vi "usrp_stream_rx.vi"() -> ()   [LabVIEW 2014]
uses:
  <vilib>/addons/Modulation/Analog/support/mod_Set Error Source.vi
  <vilib>/addons/Modulation/Digital/Support/Common/Validators/mod_Generate Filter Coefficients Validate.vi
  <vilib>/addons/Modulation/Digital/General/subVIs/mod_Generate Filter Coefficients.vi
  <vilib>/imath/engines/lvmath2/RunTimeEngine/NodeEndStatement/NIMS_NodeEndStatement_Output.vi
  <instcachedir>/0/NIMS_NodeEndStatement_Output_53EC0D466D134D7ABD903AC30B43404B.lvgen/NIMS_NodeEndStatement_Output_53EC0D466D134D7ABD903AC30B43404B_001.vi
  <vilib>/imath/engines/lvmath2/RunTimeEngine/ErrorHandling/NIMS_Finalize Error.vi
  <instrlib>/niUSRP/niUSRP Fetch Rx Data (CDB Cluster).vi
  <vilib>/addons/Modulation/niDMT.lvlib
panel:
  out "error out":errorcluster
  in  "DPSK arity":enum16{"binary", "quadrature"}(ring)=enum."quadrature"
  in  "loop bandwidth":dbl=0.0314
  in  "nfilts":i32=32
  in  "pulse shaping samples per symbol (4)":i32=4
  out "Constellation Graph":cdb[](graph)
  in  "number of samples":i64=20000
  in  "stop":bool
  in  "Timebase Clock Source":string(combo)="Internal"
  in  "Frequency Source":string(combo)="Internal"
  in  "Enabled Channels":string(combo)="0"
  in  "Active Channel":string="0"
  out "coerced gain":dbl=10.0 format="%#_6f"
  out "coerced carrier frequency":dbl=915000000.0 format="%#_6p"
  out "coerced IQ rate":dbl=1000000.0 format="%#_6p"
  in  "active antenna":string="RX2"
  in  "gain":dbl=10.0 format="%#_6f"
  in  "carrier frequency":dbl=915000000.0 format="%#_6p"
  in  "IQ rate":dbl=1000000.0 format="%#_6p"
  in  "device names":refnum<k15>="192.168.10.4"
  # "This is a usrp point-to-point communication link prototype\ndeveloped by Teng-Hui Huang, \nNetwork Information and Communications Laboratory, NTU Taiwan\nThis is the receiver program for USRP streaming mode\n\nQuick start:\n1. Connect USRPs to PC\n2. Run \"usrp_stream_tx.vi\"\n3. Run \"usrp_stream_rx.vi\"\n\nIf no error occur, you will see DPSK symbols on constellation graph\nFor any issues, please send me an e-mail\nhui811116@outlook.com\n\nThanks\nTeng-Hui Huang."
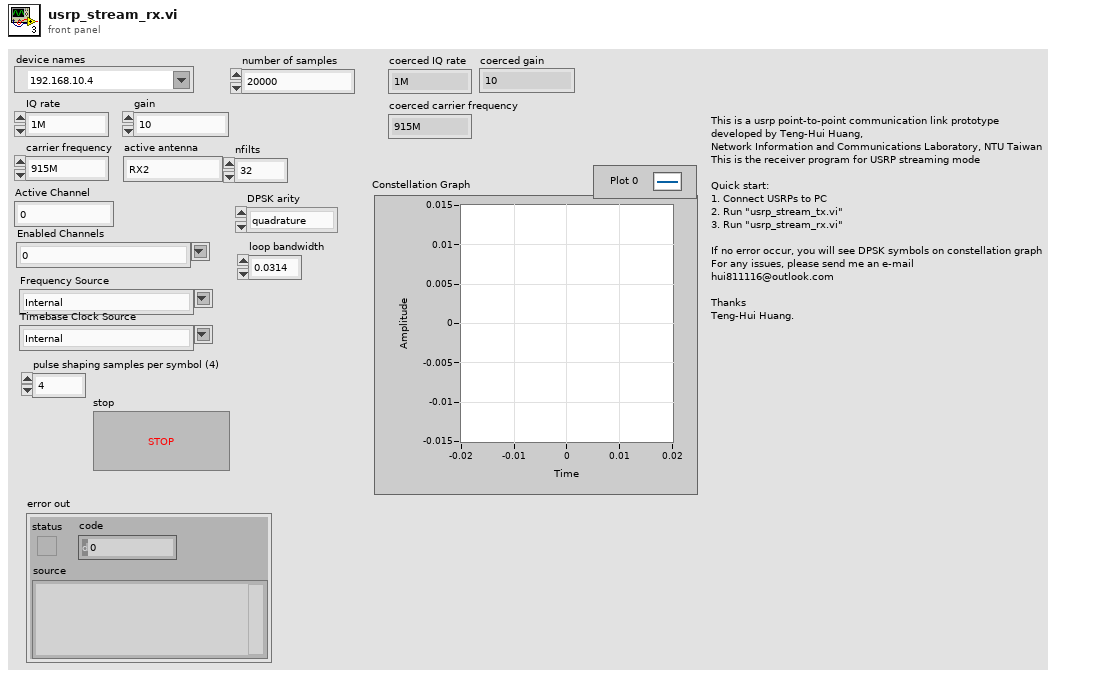
[diagram p1: front panel]
types:
  T1 = enum16{"none", "Raised Cosine", "Root Raised Cos", "Gaussian"}
  T2 = enum16{"FSK", "PSK", "QAM", "MSK", "PAM", "ASK", "CPM"}
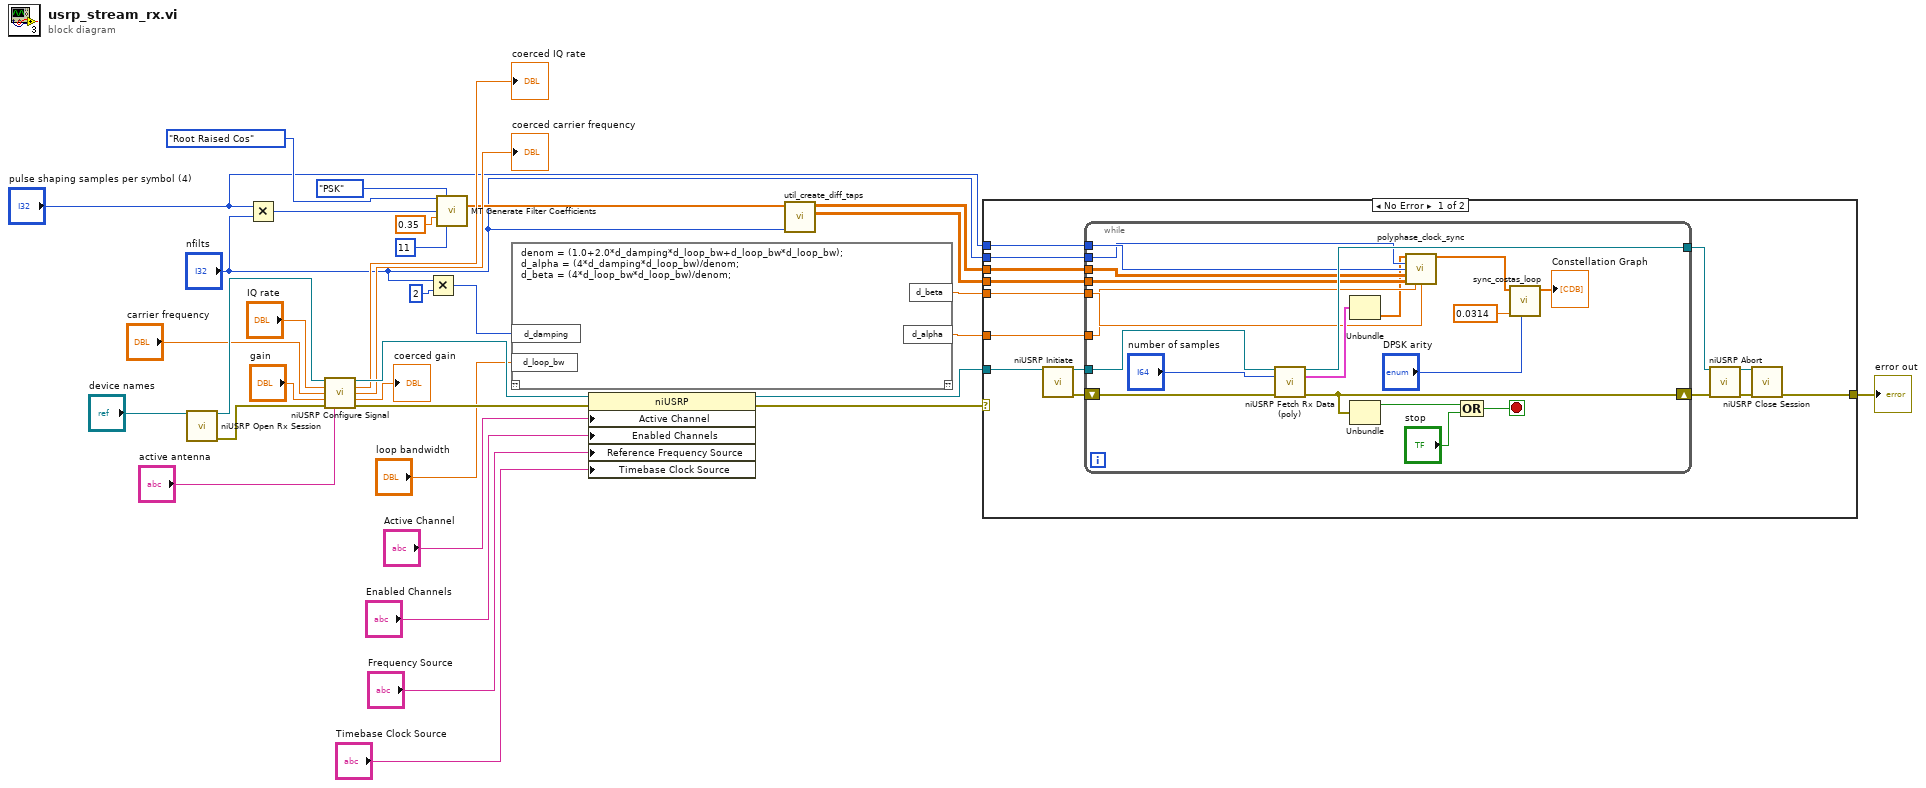
[diagram p0: block diagram]
diagram:
  n1 = call <instrlib>:"niUSRP Open Rx Session.vi"("device names"="device names") -> ("session handle out"=w31:refnum<k15>, "error out"=w30:errorcluster)  [unwired: 13 in]
  n2 = Multiply(x="pulse shaping samples per symbol (4)", y="nfilts") -> (x*y=w2:i32)
  n3 = call <instrlib>:"niUSRP Configure Signal.vi"("session handle"=w31, "IQ rate"="IQ rate", "carrier frequency"="carrier frequency", "gain"="gain", "error in (no error)"=w30, "active antenna"="active antenna") -> ("session handle out"=w33:refnum<k15>, "coerced IQ rate"=→"coerced IQ rate":dbl, "coerced carrier frequency"=→"coerced carrier frequency":dbl, "coerced gain"=→"coerced gain":dbl, "error out"=w32:errorcluster)  [unwired: 5 in]
  n4 = Multiply(x="nfilts", y=2) -> (x*y=w8:i32)
  n5 = call <vilib>:"MT Generate Filter Coefficients.vi"("pulse shaping filter (none)"=T1."Root Raised Cos", "modulation type"=T2."PSK", "matched samples per symbol (16)"=w2, "filter parameter"=0.35, "filter length (symbols)"=11) -> ("matched filter coefficients"=w12:dbl[])  [unwired: 8 in, 2 out]
  n6 = mathscript code="denom = (1.0+2.0*d_damping*d_loop_bw+d_loop_bw*d_loop_bw);\nd_alpha = (4*d_damping*d_loop_bw)/denom;\nd_beta = (4*d_loop_bw*d_loop_bw)/denom;"("d_damping"=w8, "d_loop_bw"="loop bandwidth") -> ("d_alpha"=w5:dbl, "d_beta"=w6:dbl)  [unwired: 1 in, 1 out]
  n7 = property class="niUSRP"(reference=w33, error in=w32, "Active Channel"="Active Channel", "Enabled Channels"="Enabled Channels", "Reference Frequency Source"="Frequency Source", "Timebase Clock Source"="Timebase Clock Source") -> (reference out=w17:refnum<k15>, error out=w18:errorcluster)
  n8 = call "util_create_diff_taps.vi"("nfilts"="nfilts", "taps"=w12) -> ("out diff taps"=w10:dbl[][], "out taps"=w11:dbl[][])  [unwired: 7 in, 1 out]
  n9 = case shown="No Error" w18 {
    selector: w18 -> [_ w69]
    tunnel: w17 -> [w48 _]
    tunnel: "pulse shaping samples per symbol (4)" -> [w41 _]
    tunnel: "nfilts" -> [w40 _]
    tunnel: w11 -> [w39 _]
    tunnel: w10 -> [w38 _]
    tunnel: w6 -> [w37 _]
    tunnel: w5 -> [w36 _]
    tunnel: [w35 w69] -> w1
    frame No Error {
      n10 = call <instrlib>:"niUSRP Initiate.vi"("session handle"=w48) -> ("session handle out"=w46:refnum<k15>, "error out"=w45:errorcluster)  [unwired: 13 in]
      n11 = while {
        tunnel: [w68] -> w47
        tunnel: w46 -> [w67]
        shift-right: [w53] -> w44
        shift-left: w45 -> [w66]
        tunnel: w41 -> [w63]
        tunnel: w40 -> [w62]
        tunnel: w39 -> [w61]
        tunnel: w38 -> [w60]
        tunnel: w37 -> [w59]
        tunnel: w36 -> [w58]
        stop <- w50 stop-if-true
        n12 = call-poly <instrlib>:"niUSRP Fetch Rx Data (poly).vi"("session handle"=w67, "number of samples"="number of samples", "error in (no error)"=w66) -> ("session handle out"=w68:refnum<k15>, "data"=w64:cluster{"t0":dbl, "dt":dbl, "Y":cdb[]}, "error out"=w53:errorcluster)  [unwired: 9 in, 1 out]
        n13 = Unbundle(w64) -> ("Y"=w49:cdb[])  [unwired: 2 out]
        n14 = Unbundle(w53) -> ("status"=w52:bool)  [unwired: 2 out]
        n15 = call "polyphase_clock_sync.vi"("samples"=w49, "nfilts"=w62, "sps"=w63, "taps"=w61, "diff taps"=w60, "alpha"=w58, "beta"=w59) -> ("out symbols"=w57:cdb[])  [unwired: 7 in, 1 out]
        n16 = Compound Arithmetic op=OR(w52, "stop") -> (w50:bool)
        n17 = call "sync_costas_loop.vi"("arity"="DPSK arity", "loop bandwidth"=0.0314, "symbols"=w57) -> ("outputs"=→"Constellation Graph":cdb[])  [unwired: 8 in]
      }
      n18 = call <instrlib>:"niUSRP Abort.vi"("session handle"=w47, "error in (no error)"=w44) -> ("session handle out"=w43:refnum<k15>, "error out"=w42:errorcluster)  [unwired: 12 in]
      n19 = call <instrlib>:"niUSRP Close Session.vi"("session handle"=w43, "error in (no error)"=w42) -> ("error out"=w35:errorcluster)  [unwired: 13 in]
    }
    frame Error {
    }
  }
  "error out" <- w1
